vi "lidarTrim.vi"(7 "r값 문자열":string, 8 "y+":i32, 9 "y-":i32, 10 "x+":i32, 11 "x-":i32) -> (3 "trim된xy":cluster{"x":dbl, "y":dbl}[](array[cluster]))   [LabVIEW 2015]
panel:
  out "r, theta 초기 클러스터":cluster{u32, dbl}[](array[cluster])
  out "r(mm)":u32[](array[numeric])
  out "Theta 0:180:0.5":dbl[](array[numeric])
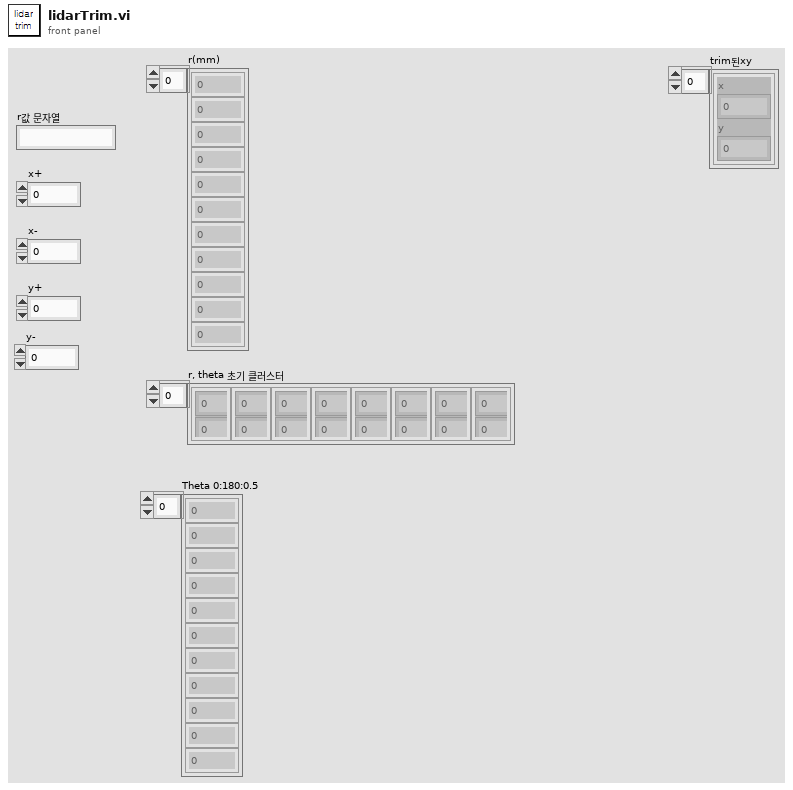
[diagram p1: front panel]
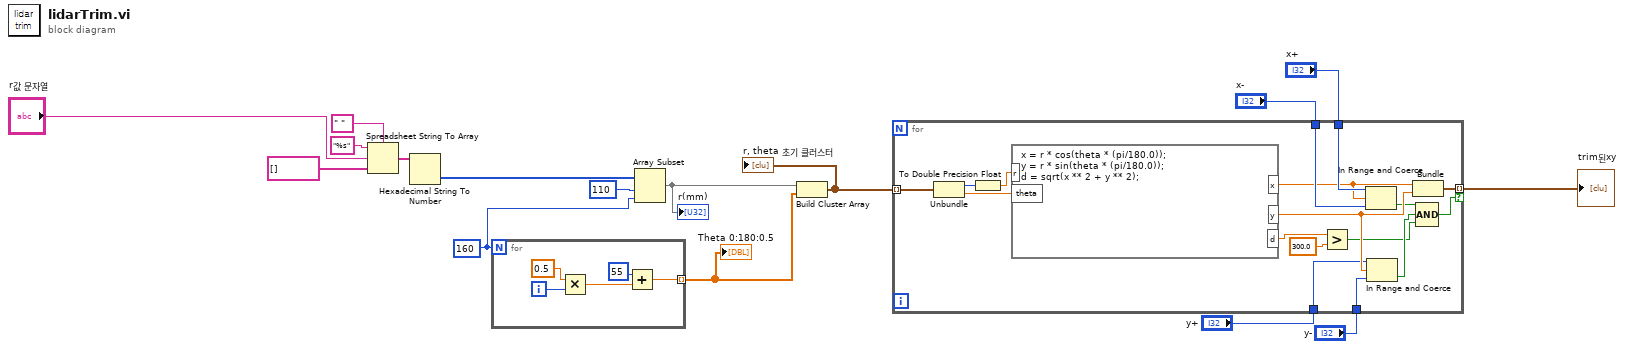
[diagram p0: block diagram]
diagram:
  w1 = 160
  n1 = Spreadsheet String To Array(delimiter (Tab)=" " ("구분 문자 (탭)"), format string="%s" ("포맷 문자열"), spreadsheet string="r값 문자열", array type (2D Dbl)=string[] [] ("배열 2")) -> (array=w5:string[])
  n2 = Hexadecimal String To Number(string=w5) -> (number=w3:u32[])  [unwired: 2 in, 1 out]
  n3 = for {
    N: w1 -> [_]
    tunnel: [w17] -> w9 mode=indexing
    i -> [w21]
    n4 = Multiply(x=0.5, y=w21) -> (x*y=w19:dbl)
    n5 = Add(x=55, y=w19) -> (x+y=w17:dbl)
  }
  "Theta 0:180:0.5" <- w9
  n6 = Array Subset(array=w3, index=110 ("인덱스"), length=w1) -> (w11:u32[])
  "r(mm)" <- w11
  n7 = Build Cluster Array(w11, w9) -> (w10:cluster{u32, dbl}[])
  "r, theta 초기 클러스터" <- w10
  n8 = for {
    tunnel: w10 -> [w38] mode=indexing
    tunnel: [w37] -> w16 mode=indexing if=w23
    tunnel: "x+" -> [w31]
    tunnel: "x-" -> [w30]
    tunnel: "y-" -> [w27]
    tunnel: "y+" -> [w26]
    n9 = Unbundle(w38) -> (w35:u32, w36:dbl)
    n10 = To Double Precision Float(number=w35) -> (double precision float=w34:dbl)
    n11 = formula code="x = r * cos(theta * (pi/180.0));\ny = r * sin(theta * (pi/180.0));\nd = sqrt(x ** 2 + y ** 2);"("r"=w34, "theta"=w36) -> ("x"=w29:dbl, "y"=w28:dbl, "d"=w32:dbl)
    n12 = Greater?(x=w32, y=300.0) -> (0:w22:bool)
    n13 = In Range and Coerce(upper limit=w31, x=w29, lower limit=w30) -> (In Range?=w25:bool)  [unwired: 1 out]
    n14 = In Range and Coerce(upper limit=w26, x=w28, lower limit=w27) -> (In Range?=w24:bool)  [unwired: 1 out]
    n15 = Bundle("x"=w29, "y"=w28) -> (w37:cluster{"x":dbl, "y":dbl})  [unwired: 1 in]
    n16 = Compound Arithmetic op=AND ("복합 연산")(w25, w24, w22) -> (w23:bool)
  }
  "trim된xy" <- w16
